vi "SR430 Error Message.vi"(0 "type of dialog (no dialog: 0)":u16(ring) items=["no dialog", "OK message", "continue or stop message"], 2 "addMessageToSource":bool, 5 "error in (no error)":errorcluster) -> (14 "message":string=" INSTRUCTIONS:\r\rNormal Use:  When using subVIs that incorporate the error in/error out (or error I/O) structure, place this handler where you want to inform the user of an error, typically at the end of the I/O data path, as the last action of the program.  If the error in error? is ERROR, the handler creates a message describing the error and its source.  If the type of dialog = 1 (default), the message is displayed to the user, who can only acknowledge it.  If the type = 2, the user can acknowledge the message or abort execution; aborting a program with active I/O is not recommended.  If the type = 0, no message is displayed; this is used to process the error programmatically, and the error out cluster elements are wired to individual terminals for that reason.  \r\rOther Use:\n\r\nlocal testing.  To test the error code of a subVI or function that does not have the error I/O structure, you can wire its error code and a source string to the local error code and error source inputs.  If error in error? indicates no error and error code is not equal to 0, the local code and source are substituted for the error in values, and error? is set TRUE (ERROR).", 15 "codeOut":i32, 16 "isError?":bool, 19 "error out":errorcluster)   [LabVIEW 2015, in "SR430Driver.lvlib"]
doc: "Contains all the instrument-specific error codes and descriptions.\n\nIn case of an error, this VI adds the error message to the error source.\nOptionaly, an error message pops up.\n\nVI Tree for the SR430 Multi-Channel Scaler from Staford Research Systems.\n\nHistory: 24-APR-2002, Dietrich Beck\n\nCopyright (C)\nGesellschaft für Schwerionenforschung, GSI\nPlanckstr. 1\n64291 Darmstadt\nGermany\n\nContact: D.Beck@gsi.de \n\nThis program is free software; you can redistribute it and/or modify it under the terms of the \nGNU General Public License as published by the Free Software Foundation; either version 2 of the license, or (at your option) any later version.\n\nThis program is distributed in the hope that it will be useful, but WITHOUT ANY WARRANTY; without even the implied warranty of MERCHANTABILITY or FITNESS FOR A PARTICULAR PURPOSE. See the GNU General License for more details (http://www.gnu.org).\n\nGesellschaft für Schwerionenforschung, GSI\nPlanckstr. 1, 64291 Darmstadt, Germany\nFor all questions and ideas contact: M.Richter@gsi.de, K.Poppensieker, H.Brand@gsi.de or D.Beck@gsi.de.\nLast update: 11-APR-2002"
uses:
  SR430Driver.lvlib
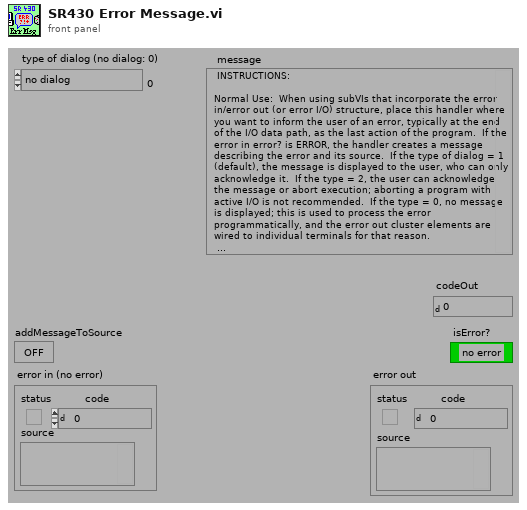
[diagram p1: front panel]
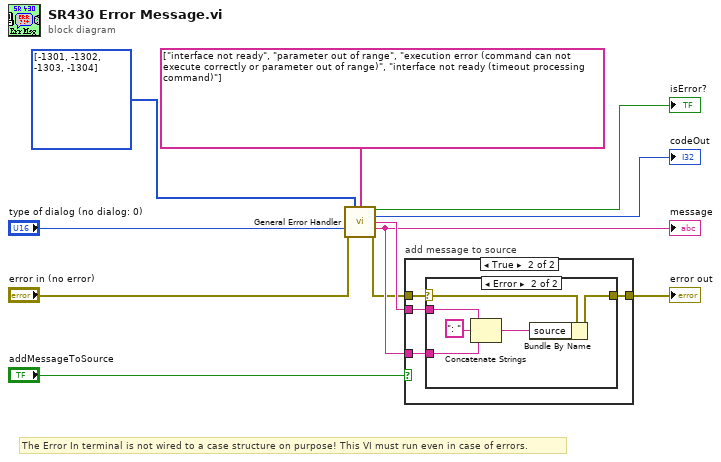
[diagram p0: block diagram]
diagram:
  # "The Error In terminal is not wired to a case structure on purpose! This VI must run even in case of errors."
  n1 = call <vilib>:"General Error Handler.vi"("[user-defined codes]"=i32[] [-1301, -1302, -1303, -1304], "[user-defined descriptions]"=string[] ["interface not ready", "parameter out of range", "execution error (command can not execute correctly or parameter out of range)", "interface not ready (timeout processing command)"], "type of dialog (OK msg:1)"="type of dialog (no dialog: 0)", "error in (no error)"="error in (no error)") -> ("error?"=→"isError?":bool, "code out"=→"codeOut":i32, "source out"=w6:string, "message"=w5:string, "error out"=w1:errorcluster)  [unwired: 7 in]
  "message" <- w5
  n2 = case "add message to source" shown="True" "addMessageToSource" {
    tunnel: [w12 w16] -> w10
    tunnel: w6 -> [_ w15]
    tunnel: w5 -> [_ w14]
    tunnel: w1 -> [w12 w13]
    frame False {
    }
    frame True {
      n3 = case shown="Error" w13 {
        selector: w13 -> [w17 w18]
        tunnel: [w17 w23] -> w16
        tunnel: w15 -> [_ w22]
        tunnel: w14 -> [_ w21]
        frame No Error {
        }
        frame Error {
          n4 = Concatenate Strings(w22, ": " ("Substring"), w21) -> (w19:string)
          n5 = Bundle By Name(cluster=w18, "source"=w19) -> (w23:errorcluster)
        }
      }
    }
  }
  "error out" <- w10
